vi "Read Molbloc Average Pressure.vi"(8 "error in (no error)":errorcluster, 11 "VISA resource name":refnum<visa-resource-name>) -> (0 "error out":errorcluster, 2 "Molbloc Average Pressure":dbl, 3 "VISA resource name out":refnum<visa-resource-name>)   [LabVIEW 2023, in "Fluke Molbox 1 Plus.lvlib"]
doc: "Read the next molbloc average pressure. The pressure value is read in the current pressure units. It is the average of the atare corrected upstream and the downstream transducers. The data string also contains flow ready information, and the pressure units."
uses:
  Fluke Molbox 1 Plus.lvlib
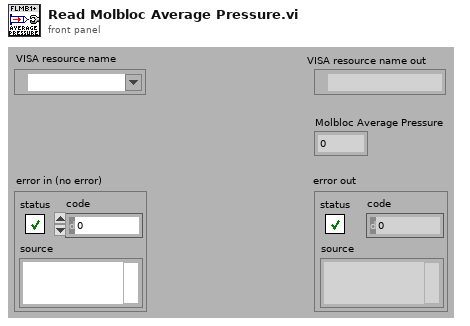
[diagram p1: front panel]
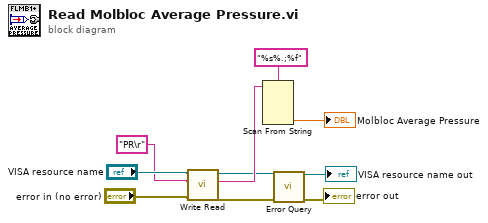
[diagram p0: block diagram]
diagram:
  n1 = call "Write Read.vi"("error in (no error)"="error in (no error)", "Write String"="PR\r" ("write buffer"), "VISA resource name"="VISA resource name") -> ("error out"=w2:errorcluster, "Read Response"=w8:string, "VISA resource name out"=w1:refnum<visa-resource-name>)  [unwired: 6 in]
  n2 = Scan From String(format string="%s%.;%f", input string=w8) -> (output 2=→"Molbloc Average Pressure":dbl)  [unwired: 5 in, 3 out]
  n3 = call "Error Query.vi"("error in (no error)"=w2, "VISA resource name"=w1) -> ("error out"=→"error out":errorcluster, "VISA resource name out"=→"VISA resource name out":refnum<visa-resource-name>)  [unwired: 6 in, 2 out]
